vi "niRFUtil MT UTIL Gaussian ZFT Filter.vi"(0 "Samples Per Symbol (16)":i32=16, 5 "Filter Parameter":dbl=0.5 step=0.01 format="%.2f", 7 "Filter Length (3)":i32=3, 11 "error in (no error)":errorcluster) -> (4 "Demod Filter Taps":T1 min=0 max=127 format="%.2f", 15 "error out":errorcluster)   [LabVIEW 2015, in "niRFUtil.lvlib"]
uses:
  niRFUtil.lvlib
  Includes/niRFUtil INC Real Array.ctl
  <vilib>/Analysis/baseanly.llb/A x Vector.vi
  <vilib>/measure/masml.llb/ma_sml_Interpolation by Zero Insert (real input).vi
  <vilib>/Analysis/baseanly.llb/Real Inverse Matrix.vi
  <vilib>/Analysis/NI_AALBase.lvlib
  <vilib>/measure/NI_MAPro.lvlib
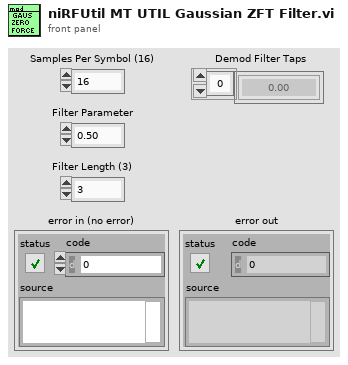
[diagram p1: front panel]
types:
  T1 = typedef "niRFUtil.lvlib/niRFUtil INC Real Array.ctl" = sgl[]
  T2 = enum32{"General", "Positive Definite", "Lower Triangular", "Upper Triangular"}
  T3 = typedef "niRFUtil.lvlib/niRFUtil INC Complex Array.ctl" = csg[]
  T4 = typedef "NI_Matrix.lvlib/RealMatrix.ctl" = dbl[][]
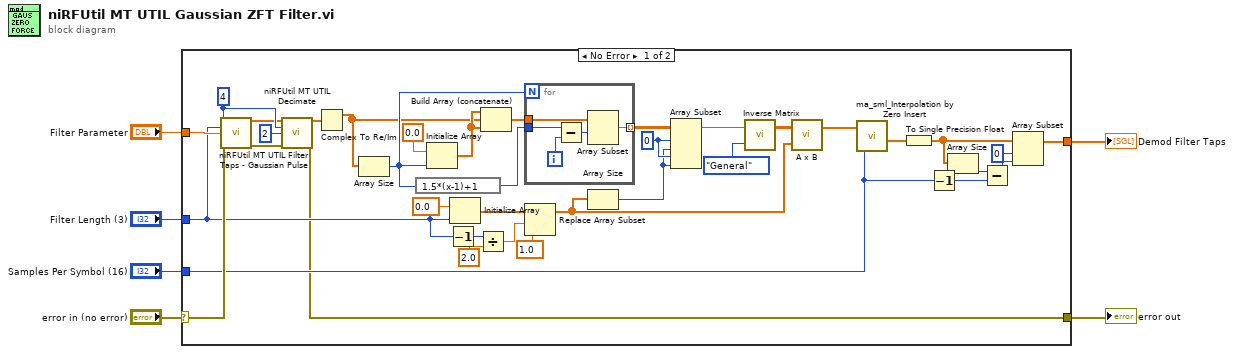
[diagram p0: block diagram]
diagram:
  n1 = case shown="No Error" "error in (no error)" {
    selector: "error in (no error)" -> [w33 w49]
    tunnel: [w9 _] -> w6
    tunnel: "Samples Per Symbol (16)" -> [w14 _]
    tunnel: "Filter Length (3)" -> [w12 _]
    tunnel: "Filter Parameter" -> [w31 _]
    tunnel: [w11 w49] -> w2
    frame No Error {
      w13 = 4
      w36 = 0 ("index")
      n2 = call "niRFUtil MT UTIL Filter Taps - Gaussian Pulse.vi"("Samples Per Symbol (16)"=w13, "Filter Length (3)"=w12, "Alpha (0.5)"=w31, "error in (no error)"=w33) -> ("Filter Coefficients"=w10:T1, "error out"=w30:errorcluster)  [unwired: 10 out]
      n3 = call "niRFUtil MT UTIL Decimate.vi"("Signal In"=w10, "Samples Per Symbol (16)"=w13, "Offset"=2, "error in (no error)"=w30) -> ("Signal Out"=w22:T3, "error out"=w11:errorcluster)  [unwired: 10 out]
      n4 = Complex To Re/Im(x + iy=w22) -> (x=w8:sgl[])  [unwired: 1 out]
      n5 = Array Size(array=w8) -> (size(s)=w34:i32)
      n6 = expression code="1.5*(x-1)+1"(w34) -> (w38:i32)
      n7 = Initialize Array(sgl 0.0, w34) -> (w39:sgl[])
      n8 = Decrement(x=w12) -> (x-1=w27:i32)
      n9 = Initialize Array(sgl 0.0 ("element"), w12) -> (w29:sgl[])
      n10 = Divide(x=w27, y=sgl 2.0) -> (x/y=w25:sgl)
      n11 = Build Array (concatenate)(w39, w8, w39) -> (w40:sgl[])
      n12 = for {
        N: w34 -> [_]
        tunnel: w40 -> [w48]
        tunnel: w38 -> [w45]
        tunnel: [w44] -> w37 mode=indexing
        i -> [w46]
        n13 = Subtract(x=w45, y=w46) -> (x-y=w47:i32)
        n14 = Array Subset(array=w48, index=w47) -> (w44:sgl[])  [unwired: 1 in]
      }
      n15 = Replace Array Subset(array=w29, new element=sgl 1.0 ("element"), index=w25) -> (w23:sgl[])
      n16 = Array Size(array=w23) -> (size(s)=w32:i32)
      n17 = Array Subset(array=w37, index (row)=w36, length (row)=w32, index (col)=w36, length (col)=w32) -> (w35:sgl[][])
      n18 = call-poly <vilib>:"Inverse Matrix.vi"("matrix type"=T2."General", "Input Matrix"=w35) -> ("Inverse Matrix"=w41:T4)  [unwired: 1 out]
      n19 = call-poly <vilib>:"A x B.vi"("Vector"=w23, "A"=w41) -> ("A x Vector"=w16:dbl[])  [unwired: 1 out]
      n20 = call-poly <vilib>:"ma_sml_Interpolation by Zero Insert.vi"("L"=w14, "x"=w16) -> ("y"=w20:dbl[])
      n21 = To Single Precision Float(number=w20) -> (single precision float=w7:sgl[])
      n22 = Decrement(x=w14) -> (x-1=w17:i32)
      n23 = Array Size(array=w7) -> (size(s)=w19:i32)
      n24 = Subtract(x=w19, y=w17) -> (x-y=w18:i32)
      n25 = Array Subset(array=w7, index=0, length=w18) -> (w9:sgl[])
    }
    frame Error {
    }
  }
  "error out" <- w2
  "Demod Filter Taps" <- w6
